vi "SLAM Main.vi"() -> ()   [LabVIEW 2009]
uses:
  <vilib>/Analysis/Matrix/Datatypes/RealMatrix.ctl
  <vilib>/Platform/TimedLoop/XDataNode/XDataNode.xnode
  <vilib>/Platform/TimedLoop/XDataNode/loadlvalarms.vi
  <vilib>/Platform/TimedLoop/XDataNode/timing_clust.ctl
  <vilib>/Platform/TimedLoop/XDataNode/nitl_modes.ctl
  <vilib>/Platform/TimedLoop/XDataNode/wakeup.ctl
  <vilib>/Platform/TimedLoop/XDataNode/XDNodeRunTimeDep.lvlib
  <vilib>/Analysis/Matrix/NI_Matrix.lvlib
panel:
  out "Kalman Estimate Matrices.X":T1
  out "XY Graph 3":cluster{dbl[], dbl[]}(graph)
  out "XY Graph 2":cluster{dbl[], dbl[]}[](graph)
  out "XY Graph":cluster{dbl[], dbl[]}[](graph)
  out "error out":errorcluster={"status"=FALSE, "code"=1073676294, "source"="VISA Read in Get Distance.vi->CREATE FG.vi->SLAM Main.vi"}
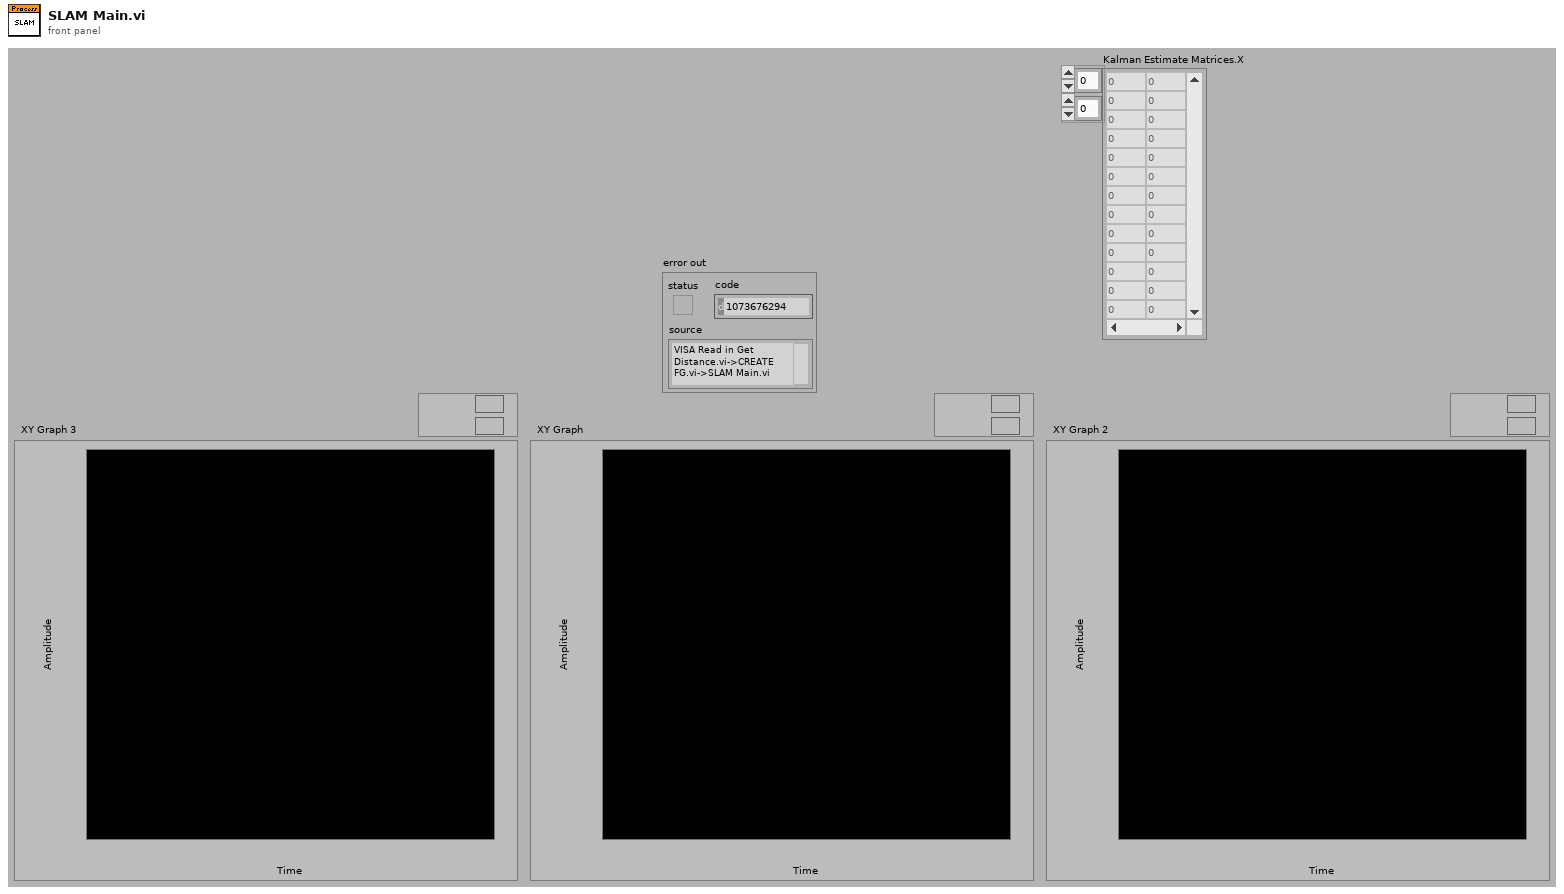
[diagram p1: front panel]
types:
  T1 = typedef "NI_Matrix.lvlib/RealMatrix.ctl" = dbl[][]
  T2 = typedef "XDNodeRunTimeDep.lvlib/timing_clust.ctl" = cluster{"Expected End [f-1]":u64, "Actual End [f-1]":u64, "Finished Late? [f-1]":bool, "Expected End [i-1]":u64, "Actual End [i-1]":u64, "Finished Late? [i-1]":bool, "Expected Start [i]":u64, "Actual Start [i]":u64, "Expected Start [f]":u64, "Actual Start [f]":u64, "Source Name":string, "Structure Name":string, "Period":i64, "Deadline":i64, "Offset":i64, "Start":i64, "Priority":i32, "Timeout":i32, "Mode":T3, "Wakeup Reason":T4, "Error":errorcluster, "Source Type":string, "Secondary Source Type":string, "Global End Time":u64, "Global Start Time":u64, "Frame Duration":u64, "Iteration Duration":u64, "Assigned CPU":i32, "I/O Scan Engine Mode":u32}
  T3 = typedef "XDNodeRunTimeDep.lvlib/nitl_modes.ctl" = enum32{"No Change", "Process missed periods, maintain original phase", "Discard missed periods, maintain original phase", "Process missed periods, ignore original phase", "Discard missed periods, ignore original phase"}
  T4 = typedef "XDNodeRunTimeDep.lvlib/wakeup.ctl" = enum32{"Normal", "Aborted", "Asynchronous wakeup", "Timing source error", "Timed loop error", "Timeout"}
  T5 = typedef "SLAM.ctl" = cluster{"Landmark Array":cluster{"ID":dbl, "X_Position_Estimate":dbl, "Y_Position_Estimate":dbl, "Covariance Matrix":T1}[], "System Matrices":cluster{"F":T1, "G":T1, "H":T1, "V":T1, "W":T1, "K":T1}, "Kalman Estimate Matrices":cluster{"X":T1, "P":T1}, "LM ID's":dbl[]}
  T6 = cluster{"X Array":dbl[], "Best Polynomial Fit":dbl[]}[]
  T7 = cluster{"ID":dbl, "X_Position_Estimate":dbl, "Y_Position_Estimate":dbl, "Covariance Matrix":T1}[]
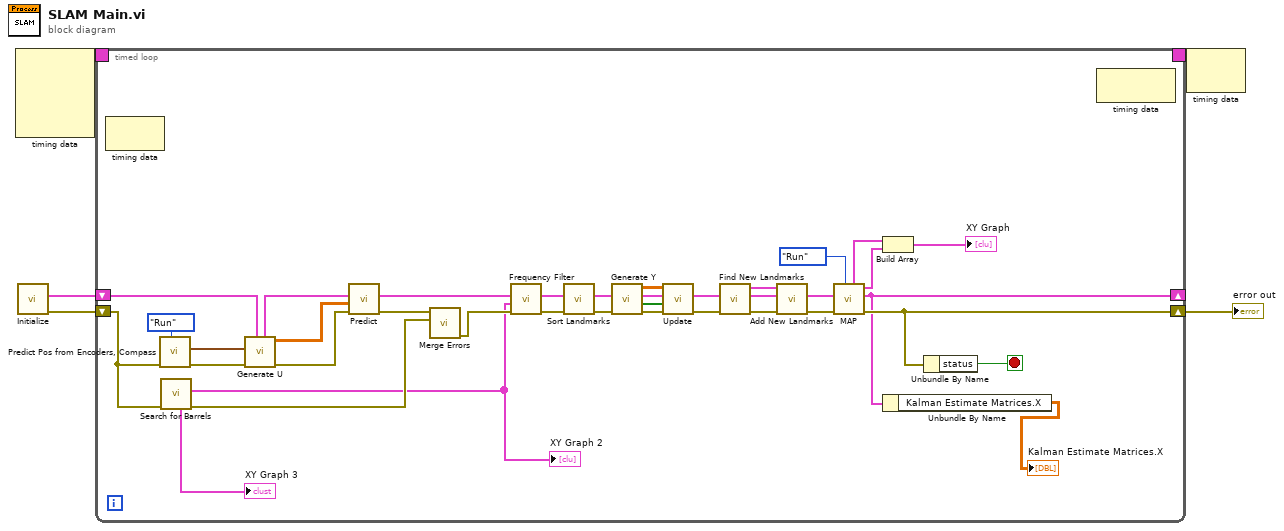
[diagram p0: block diagram]
diagram:
  n1 = node-c288() -> (w5:T2)  [unwired: 4 in]
  n2 = call "Initialize.vi"() -> ("error out"=w2:errorcluster, "SLAM Out"=w3:T5)  [unwired: 10 in]
  n3 = timed-loop {
    timing: w5 -> [_]
    timing-out: [_] -> w4
    shift-right: [w12] -> _
    shift-left: w3 -> [w41]
    shift-right: [w23] -> w1
    shift-left: w2 -> [w19]
    stop <- w15 stop-if-true
    n4 = node-c288() -> ()  [unwired: 1 in, 1 out]
    n5 = call "Predict Pos from Encoders, Compass.vi"("Cmd"=enum16{"Init", "Run"}."Run", "error in (no error)"=w19) -> ("error out"=w21:errorcluster, "XYT"=w20:cluster{"X":dbl, "Y":dbl, "Theta":dbl})  [unwired: 8 in]
    n6 = call "Search for Barrels.vi"("error in (no error)"=w19) -> ("error out"=w18:errorcluster, "Observed LM Array"=w6:T6, "RAW SICK"=→"XY Graph 3":cluster{dbl[], dbl[]})  [unwired: 8 in]
    "XY Graph 2" <- w6
    n7 = call "Generate U.vi"("SLAM In"=w41, "error in (no error)"=w21, "XYT"=w20) -> ("error out"=w42:errorcluster, "U"=w28:T1, "SLAM Out"=w40:T5)  [unwired: 6 in]
    n8 = call "Predict.vi"("error in (no error)"=w42, "U"=w28, "SLAM In"=w40) -> ("error out"=w17:errorcluster, "SLAM Out"=w9:T5)  [unwired: 7 in]
    n9 = call <vilib>:"Merge Errors.vi"("error in 2 (no error)"=w18, "error in 1 (no error)"=w17) -> ("error out"=w8:errorcluster)  [unwired: 5 in]
    n10 = call "Frequency Filter.vi"("error in (no error)"=w8, "Observed LM Array"=w6, "SLAM In"=w9) -> ("error out"=w10:errorcluster, "SLAM Out"=w7:T5)  [unwired: 7 in]
    n11 = call "Sort Landmarks.vi"("error in (no error)"=w10, "SLAM In"=w7) -> ("error out"=w36:errorcluster, "SLAM Out"=w24:T5)  [unwired: 8 in]
    n12 = call "Generate Y.vi"("error in (no error)"=w36, "SLAM In"=w24) -> ("error out"=w39:errorcluster, "Reobserved Array"=w35:bool[], "SLAM Out"=w25:T5, "Y"=w38:T1)  [unwired: 6 in]
    n13 = call "Update.vi"("error in (no error)"=w39, "Reobserved Array"=w35, "SLAM In"=w25, "Y"=w38) -> ("error out"=w37:errorcluster, "SLAM Out"=w27:T5)  [unwired: 6 in]
    n14 = call "Find New Landmarks.vi"("error in (no error)"=w37, "SLAM In"=w27) -> ("error out"=w34:errorcluster, "SLAM Out"=w33:T5, "New LM's"=w32:T7)  [unwired: 7 in]
    n15 = call "Add New Landmarks.vi"("error in (no error)"=w34, "SLAM In"=w33, "New LM's"=w32) -> ("error out"=w31:errorcluster, "SLAM Out"=w26:T5)  [unwired: 7 in]
    n16 = call "MAP.vi"("Cmd"=enum16{"Init", "Run"}."Run", "error in (no error)"=w31, "SLAM In"=w26) -> ("error out"=w23:errorcluster, "SLAM Out"=w12:T5, "Landmark Array"=w16:cluster{dbl[], dbl[]}, "Robot Position"=w29:cluster{dbl[], dbl[]})  [unwired: 5 in]
    n17 = Build Array(w29, w16) -> (→"XY Graph":cluster{dbl[], dbl[]}[])
    n18 = Unbundle By Name(w12) -> ("Kalman Estimate Matrices.X"=→"Kalman Estimate Matrices.X":T1)
    n19 = Unbundle By Name(w23) -> ("status"=w15:bool)
    n20 = node-c288() -> ()  [unwired: 1 in, 1 out]
  }
  "error out" <- w1
  n21 = node-c288(w4) -> ()  [unwired: 1 out]
